vi "2D Gaussian - Function.vi"(3 "output control":T1, 4 "data":T2, 5 "X":dbl[](array[numeric]), 6 "a":dbl[](array[numeric])) -> (0 "error out":errorcluster, 1 "f'(X,a)":dbl[][](array[numeric]), 2 "f(X,a)":dbl[](array[numeric]))   [LabVIEW 2016]
doc: "This template is the starting point for creating a model function to be passed to the Nonlinear Curve Fit.vi."
uses:
  <vilib>/gmath/NumericalOptimization/objective function data.ctl
  <vilib>/gmath/NumericalOptimization/LM_output select.ctl
  <vilib>/gmath/NI_Gmath.lvlib
panel:
  # "Amp\nXo\nYo\nWx\nWy\nOffset"
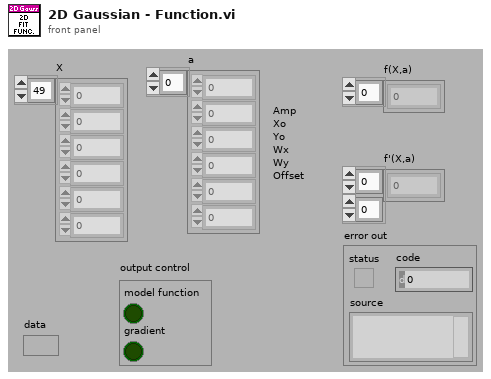
[diagram p1: front panel]
types:
  T1 = typedef "NI_Gmath.lvlib/LM_output select.ctl" = cluster{"model function":bool, "gradient":bool}
  T2 = typedef "NI_Gmath.lvlib/objective function data.ctl" = variant
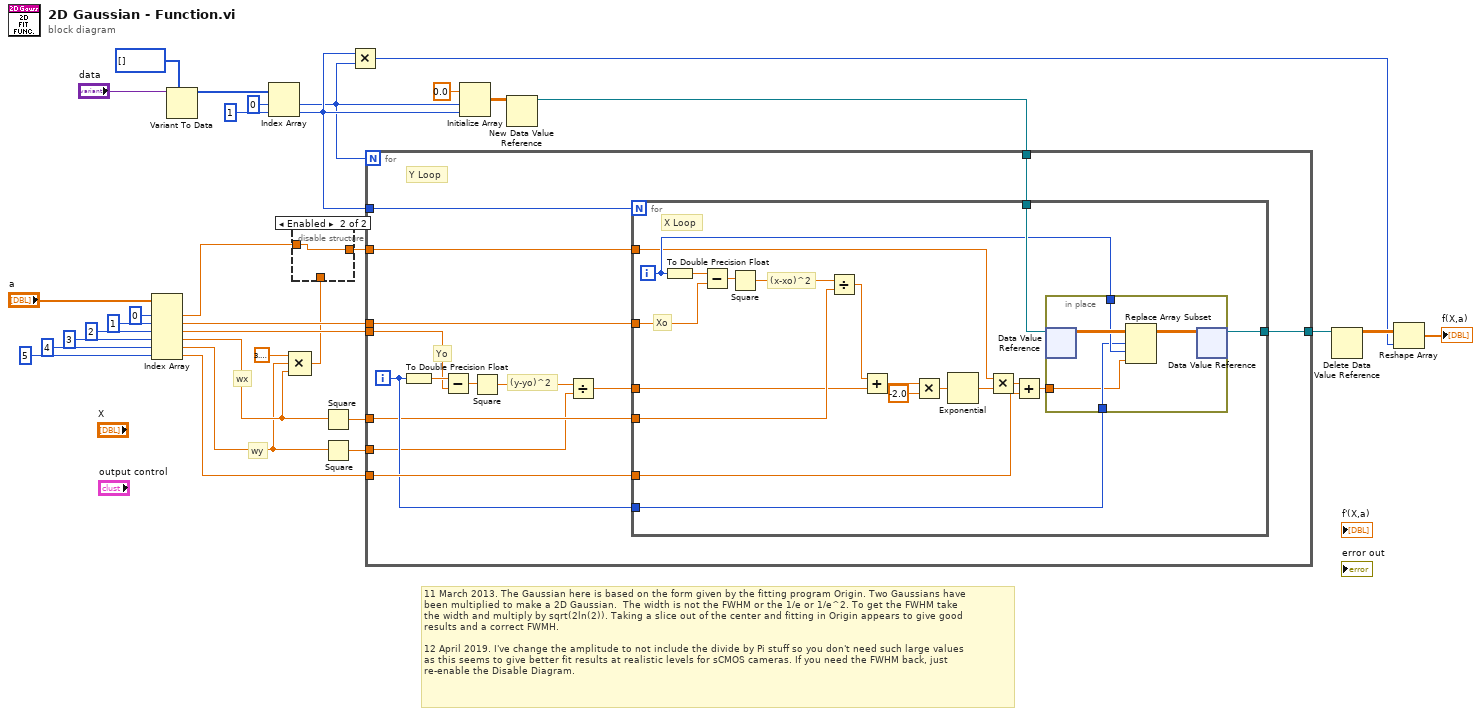
[diagram p0: block diagram]
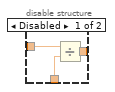
[diagram p2: hidden frame]
diagram:
  # "11 March 2013. The Gaussian here is based on the form given by the fitting program Origin. Two Gaussians have\nbeen multiplied to make a 2D Gaussian.  The width is not the FWHM or the 1/e or 1/e^2. To get the FWHM take\nthe width and multiply by sqrt(2ln(2)). Taking a slice out of the center and fitting in Origin appears to give good\nresults and a correct FWMH.\n\n12 April 2019. I've change the amplitude to not include the divide by Pi stuff so you don't need such large values\nas this seems to give better fit results at realistic levels for sCMOS cameras. If you need the FWHM back, just\nre-enable the Disable Diagram."
  # "wy"
  # "wx"
  n1 = Index Array(array="a", index #1=0 ("index"), index #2=1 ("index"), index #3=2 ("index"), index #4=3 ("index"), index #5=4 ("index"), index #6=5 ("index")) -> (element #1=w18:dbl, element #2=w31:dbl, element #3=w30:dbl, element #4=w20:dbl, element #5=w19:dbl, element #6=w29:dbl)
  n2 = Variant To Data(type=i32[] [], Variant="data") -> (data=w12:i32[])  [unwired: 1 in, 1 out]
  n3 = Index Array(array=w12, index #1=0 ("index"), index #2=1 ("index")) -> (element #1=w7:i32, element #2=w8:i32)
  n4 = Compound Arithmetic op=MULTIPLY(3.141592653589793, w19, w20) -> (w17:dbl)
  n5 = disable-structure shown="Enabled" {
    disable-tunnel: w18 -> [w35 w36]
    disable-tunnel: w17 -> [w34 _]
    disable-tunnel: [w33 w36] -> w16
    frame Disabled {
      n6 = Divide(x=w35, y=w34) -> (x/y=w33:dbl)
    }
    frame Enabled {
    }
  }
  n7 = Square(x=w20) -> (x^2=w23:dbl)
  n8 = Square(x=w19) -> (x^2=w22:dbl)
  n9 = Multiply(x=w8, y=w7) -> (x*y=w9:i32)
  n10 = Initialize Array(0.0 ("element"), w7, w8) -> (w27:dbl[][])
  n11 = New Data Value Reference(data value=w27) -> (data value reference=w26:refnum<data-value>)  [unwired: 1 in, 1 out]
  n12 = for {
    N: w7 -> [_]
    tunnel: w31 -> [w50]
    tunnel: w30 -> [w47]
    tunnel: w29 -> [w49]
    tunnel: w26 -> [w45]
    tunnel: [w43] -> w25
    tunnel: w23 -> [w42]
    tunnel: w22 -> [w40]
    tunnel: w16 -> [w38]
    tunnel: w8 -> [w37]
    i -> [w44]
    # "(y-yo)^2"
    # "Yo"
    # "Y Loop"
    n13 = To Double Precision Float(number=w44) -> (double precision float=w48:dbl)
    n14 = Subtract(x=w48, y=w47) -> (x-y=w46:dbl)
    n15 = Square(x=w46) -> (x^2=w41:dbl)
    n16 = Divide(x=w41, y=w40) -> (x/y=w39:dbl)
    n17 = for {
      N: w37 -> [_]
      tunnel: w50 -> [w68]
      tunnel: w49 -> [w66]
      tunnel: w45 -> [w65]
      tunnel: w44 -> [w63]
      tunnel: [w61] -> w43
      tunnel: w42 -> [w59]
      tunnel: w39 -> [w58]
      tunnel: w38 -> [w51]
      i -> [w64]
      # "Xo"
      # "(x-xo)^2"
      # "X Loop"
      n18 = To Double Precision Float(number=w64) -> (double precision float=w69:dbl)
      n19 = Subtract(x=w69, y=w68) -> (x-y=w67:dbl)
      n20 = Square(x=w67) -> (x^2=w60:dbl)
      n21 = Divide(x=w60, y=w59) -> (x/y=w57:dbl)
      n22 = Add(x=w57, y=w58) -> (x+y=w56:dbl)
      n23 = Multiply(x=w56, y=-2.0) -> (x*y=w54:dbl)
      n24 = Exponential(1:w54) -> (0:w53:dbl)
      n25 = Multiply(x=w51, y=w53) -> (x*y=w52:dbl)
      n26 = Add(x=w52, y=w66) -> (x+y=w62:dbl)
      n27 = in-place {
        in-place-border: w64 -> [w72]
        in-place-border: w63 -> [w71]
        in-place-border: w62 -> [w70]
        n28 = in-place-dvr #1(w65) -> (w74:dbl[][])  [unwired: 1 out]
        n29 = Replace Array Subset(array=w74, new element=w70, index (row)=w71, index (col)=w72) -> (w73:dbl[][])
        n30 = in-place-dvr #1(w73) -> (w61:refnum<data-value>)  [unwired: 1 out]
      }
    }
  }
  n31 = Delete Data Value Reference(data value reference=w25) -> (data value=w15:dbl[][])  [unwired: 1 in, 1 out]
  n32 = Reshape Array(w15, w9) -> (→"f(X,a)":dbl[])
